vi "Reading_Instrument.vi"(0 "Read String":string, 11 "error in":errorcluster) -> (4 "Readed Data":string, 15 "error out":errorcluster)   [LabVIEW 2020]
doc: "This VI will read the data stored in the .ini file with the help of keys and return this as output"
uses:
  <vilib>/Utility/config.llb/Read Key (String).vi
  <vilib>/Utility/config.llb/NI_LVConfig.lvlib
panel:
  # "This VI will read the stored data from the storage file"
  # "Command: MEASure:CURRent/VOLTage:DC"
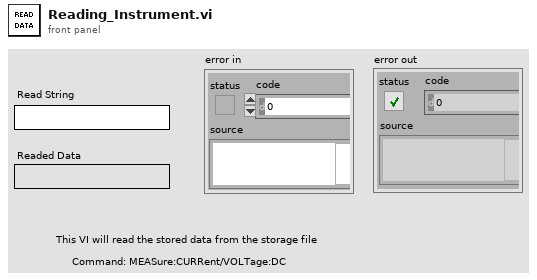
[diagram p1: front panel]
types:
  T1 = typedef "NI_LVConfig.lvlib/Config Data RefNum.ctl" = refnum<k1>
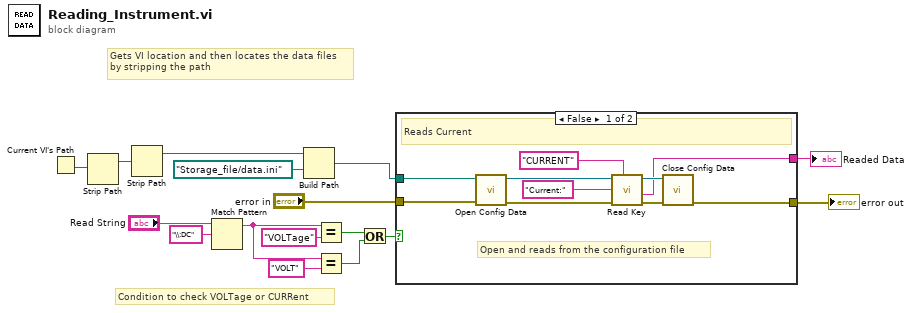
[diagram p0: block diagram]
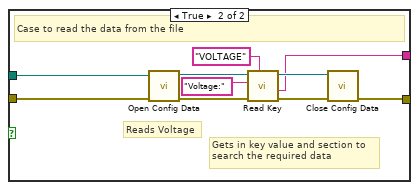
[diagram p2: hidden frame]
diagram:
  # "Condition to check VOLTage or CURRent"
  # "Gets VI location and then locates the data files\nby stripping the path"
  n1 = Current VI's Path() -> (path=w12:path)
  n2 = Strip Path(path=w12) -> (stripped path=w11:path)  [unwired: 1 out]
  n3 = Strip Path(path=w11) -> (stripped path=w10:path)  [unwired: 1 out]
  n4 = Match Pattern(string="Read String", regular expression="\\:DC") -> (before substring=w5:string)  [unwired: 1 in, 3 out]
  n5 = Build Path(base path=w10, name or relative path=path "Storage_file/data.ini") -> (appended path=w6:path)
  n6 = Equal?(x=w5, y="VOLTage") -> (x = y?=w2:bool)
  n7 = Equal?(x=w5, y="VOLT") -> (x = y?=w1:bool)
  n8 = Or(x=w2, y=w1) -> (x .or. y?=w3:bool)
  n9 = case shown="False" w3 {
    tunnel: w6 -> [w25 w27]
    tunnel: [w19 w31] -> w13
    tunnel: [w18 w29] -> w8
    tunnel: "error in" -> [w17 w28]
    frame False {
      # "Open and reads from the configuration file"
      # "Reads Current"
      n10 = call <vilib>:"Open Config Data.vi"("error in (no error)"=w17, "configuration file path"=w25) -> ("error out"=w26:errorcluster, "refnum"=w22:T1)  [unwired: 7 in, 1 out]
      n11 = call-poly <vilib>:"Read Key.vi"("section"="CURRENT", "error in (no error)"=w26, "key"="Current:", "refnum"=w22) -> ("error out"=w24:errorcluster, "value"=w19:string, "refnum out"=w23:T1)  [unwired: 4 in, 1 out]
      n12 = call <vilib>:"Close Config Data.vi"("error in (no error)"=w24, "refnum"=w23) -> ("error out"=w18:errorcluster)  [unwired: 8 in, 1 out]
    }
    frame True {
      # "Reads Voltage"
      # "Gets in key value and section to\nsearch the required data"
      # "Case to read the data from the file"
      n13 = call <vilib>:"Open Config Data.vi"("error in (no error)"=w28, "configuration file path"=w27) -> ("error out"=w35:errorcluster, "refnum"=w36:T1)  [unwired: 7 in, 1 out]
      n14 = call-poly <vilib>:"Read Key.vi"("section"="VOLTAGE", "error in (no error)"=w35, "key"="Voltage:", "refnum"=w36) -> ("error out"=w33:errorcluster, "value"=w31:string, "refnum out"=w34:T1)  [unwired: 4 in, 1 out]
      n15 = call <vilib>:"Close Config Data.vi"("error in (no error)"=w33, "refnum"=w34) -> ("error out"=w29:errorcluster)  [unwired: 8 in, 1 out]
    }
  }
  "Readed Data" <- w13
  "error out" <- w8
